vi "Singing Helmet.vi"(8 "error in (no error)":errorcluster) -> (0 "error out":errorcluster)   [LabVIEW 2020, in "MainVIs.lvlib"]
doc: "This template is for the Queued Message Handler design pattern.\n\nThe Event Handling Loop generates messages based on user interface actions.\n\nThe Message Handling Loop processes messages generated by the Event Handling Loop, or by other messages. The messages are string values, so new messages can be added easily to the Message Cases case structure in the Message Handling Loop. Each message cluster can also provide an optional value for Message Data, which is a variant that can be converted to whatever message-specific data is required."
uses:
  MainVIs.lvlib
  Collection Support/Controls/UI Data SH.ctl
  Collection Support/Controls/CollectStates.ctl
  Collection Support/Controls/FirstCall.ctl
  Collection Support/Message Queue/Enqueue Message (Single).vi
  Collection Support/Message Queue/Enqueue Message (Array).vi
  <vilib>/Utility/error.llb/Error Cluster From Error Code.vi
  <vilib>/ErrorRing/Error Ring.xnode
  Collection Support/Message Queue/Message Queue.lvlib
  Collection Support/User Event - Stop/User Event - Stop.lvlib
  CollectionSupport.lvlib
panel:
  out "Flow":dbl
  out "Pressure":dbl
  in  "Blank Button":bool
  in  "Calibrate":bool
  out "Message":string
  in  "Settings":bool
  in  "Collect":bool
  in  "Exit":bool
  out "Pressure":dynamicdata(graph)
  out "Audio Chart":dynamicdata(graph)
  out "Flow":dynamicdata(graph)
  out "All Data Collected":dynamicdata(graph)
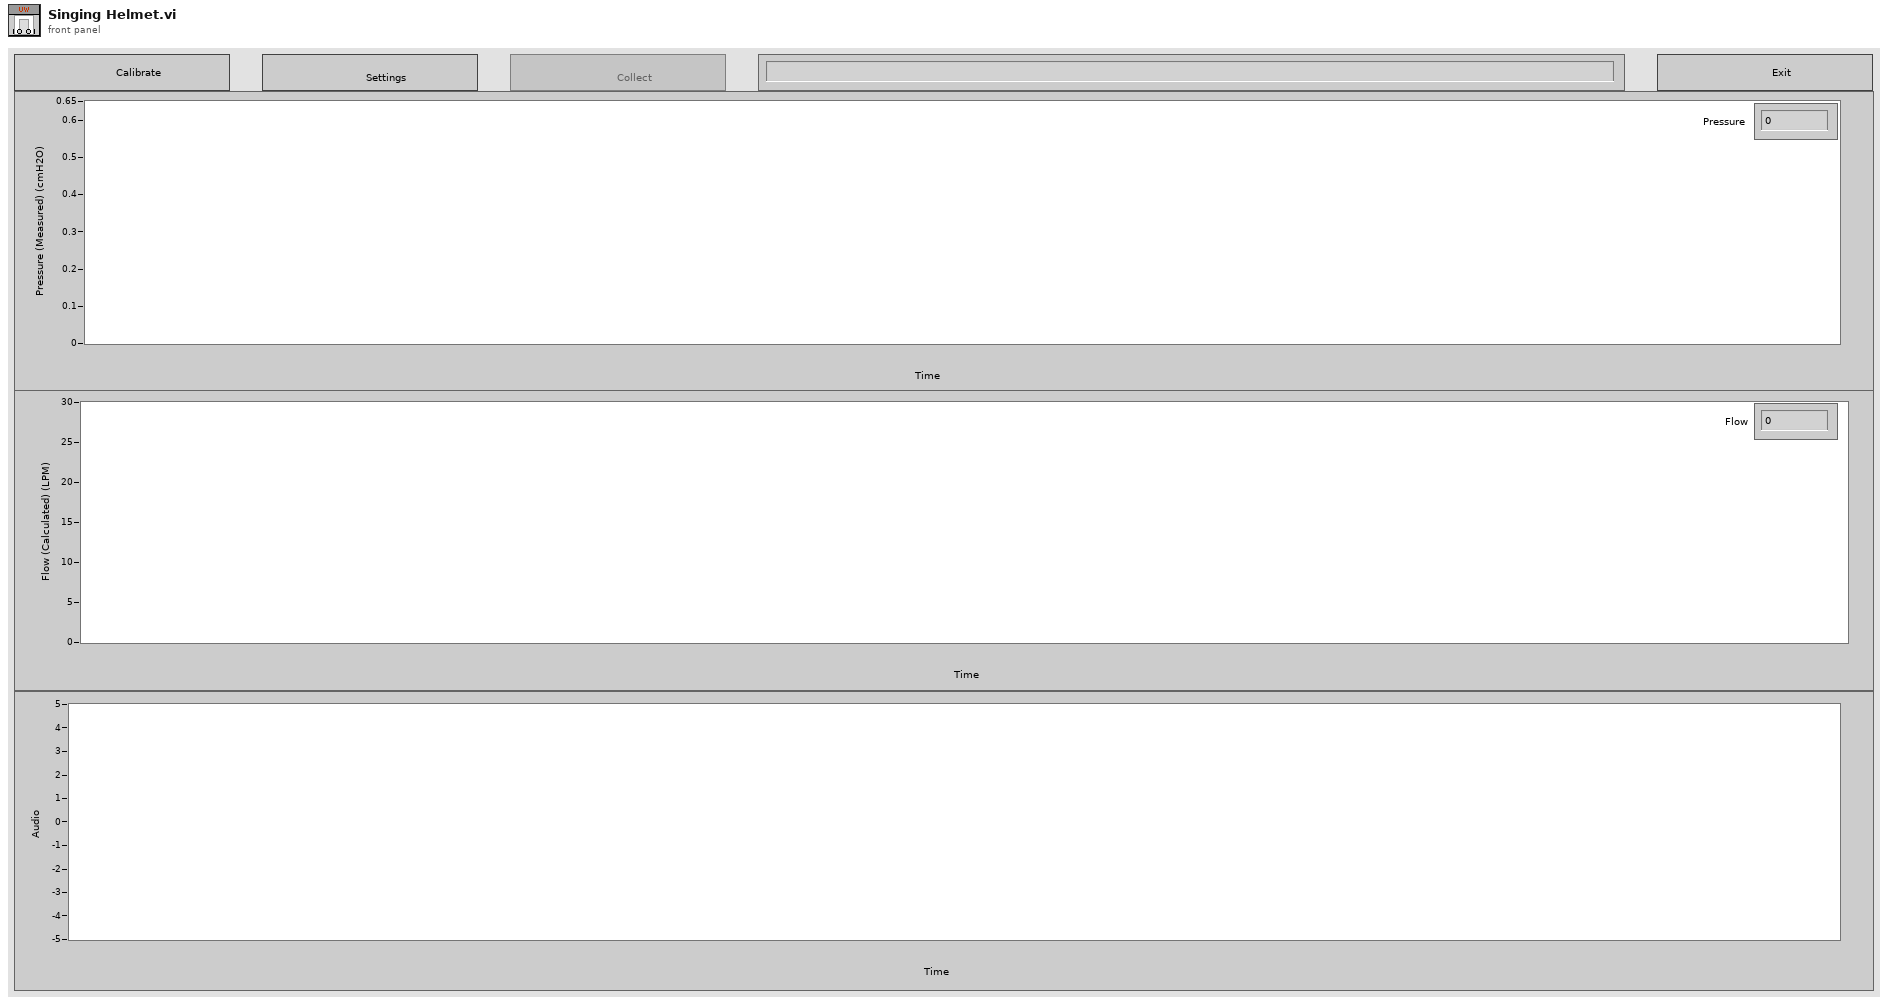
[diagram p1: front panel]
types:
  T1 = typedef "CollectionSupport.lvlib/UI Data SH.ctl" = cluster{"Message":string, "Trial":i32, "Calibrate Ref":refnum<vi>, "Collect Ref":refnum<vi>, "Exit Button Ref":refnum<vi>, "Settings Ref":refnum<vi>, "Data Display Ref":refnum<vi>, "Time":dbl, "Slope":dbl, "Intercept":dbl, "Gain":dbl, "Offset":dbl, "Task":string, "Subject":string, "Pressure":dynamicdata, "Flow":dynamicdata, "Audio Chart":dynamicdata, "Pressure/Flow":dynamicdata, "Audio Collected":dynamicdata}
  T2 = typedef "CollectionSupport.lvlib/Message Queue.lvlib/All Message Queues.ctl" = cluster{"UI":refnum<queue>}
  T3 = typedef "CollectionSupport.lvlib/CollectStates.ctl" = enum16{"Start", "Run", "Save", "Check", "Exit"}
  T4 = typedef "CollectionSupport.lvlib/FirstCall.ctl" = enum16{"First", "After"}
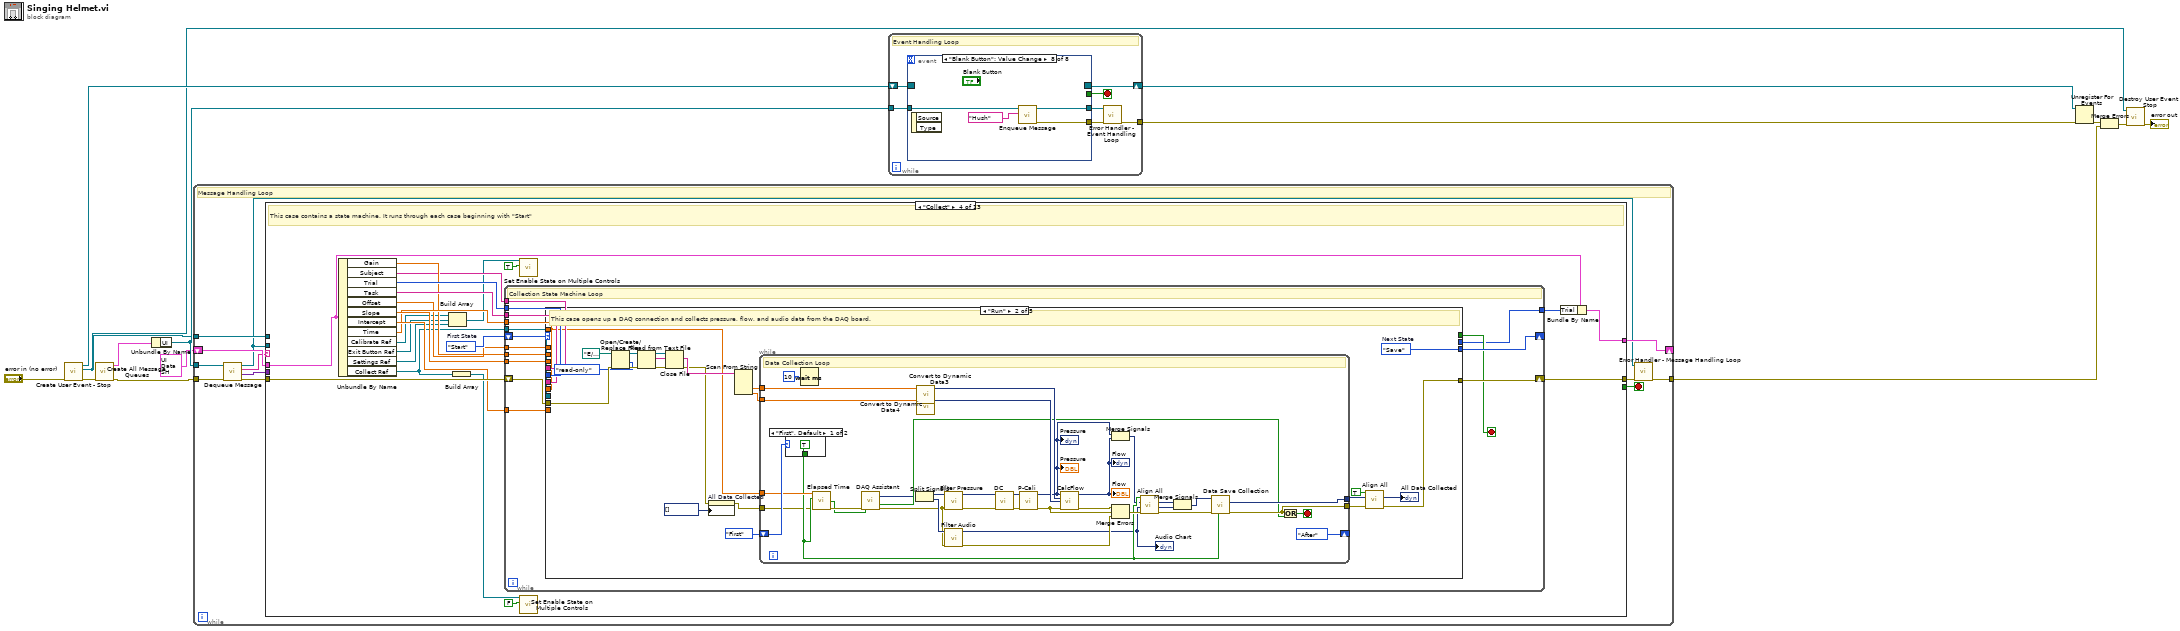
[diagram p0: block diagram]
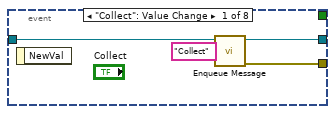
[diagram p2: hidden frame]
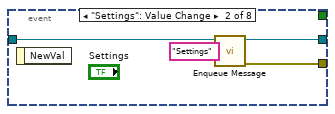
[diagram p3: hidden frame]
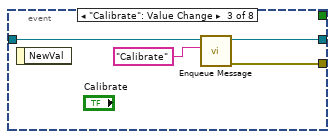
[diagram p4: hidden frame]
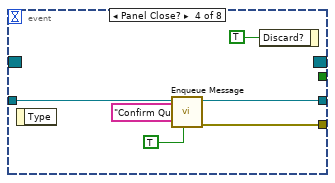
[diagram p5: hidden frame]
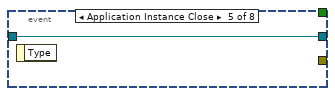
[diagram p6: hidden frame]
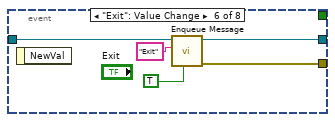
[diagram p7: hidden frame]
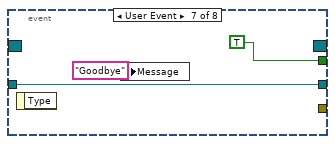
[diagram p8: hidden frame]
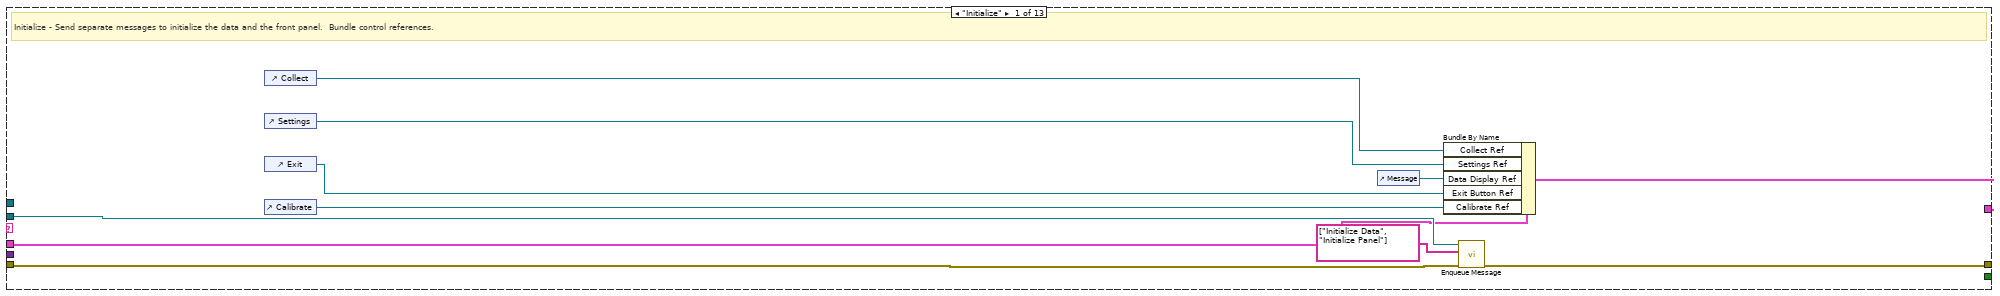
[diagram p9: hidden frame]
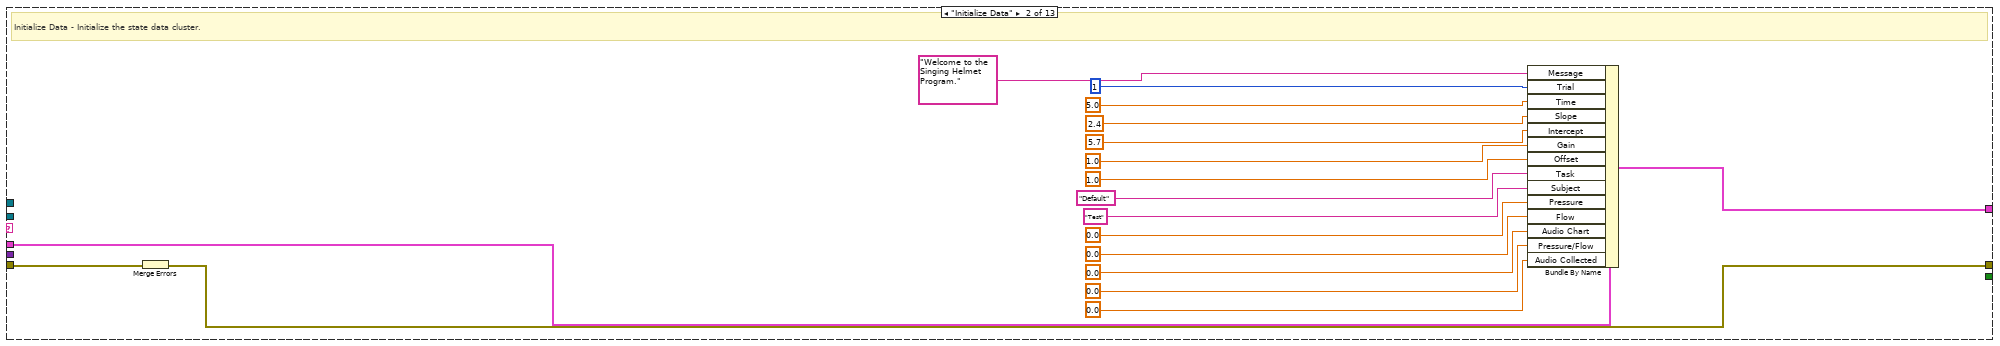
[diagram p10: hidden frame]
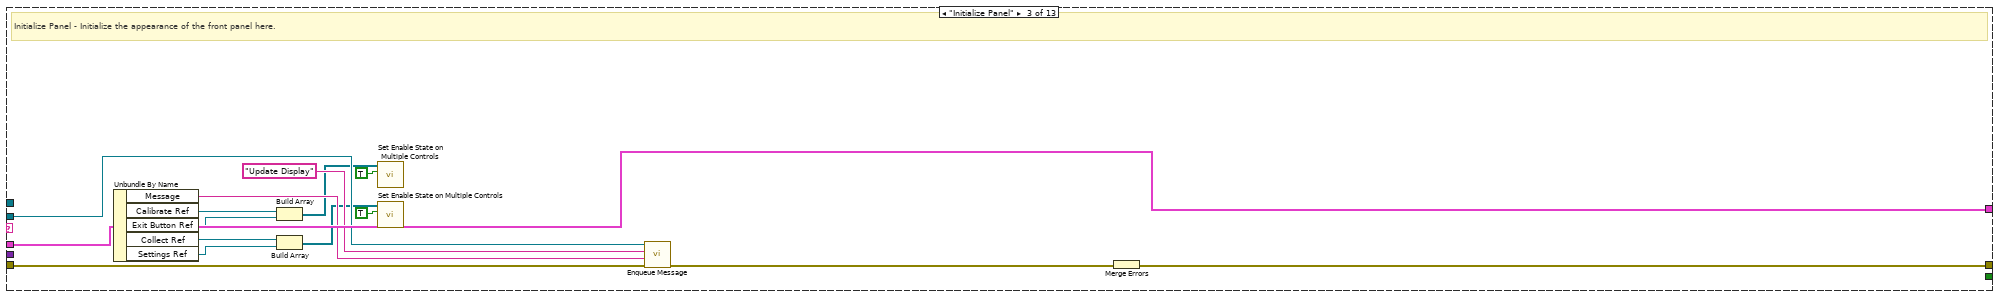
[diagram p11: hidden frame]
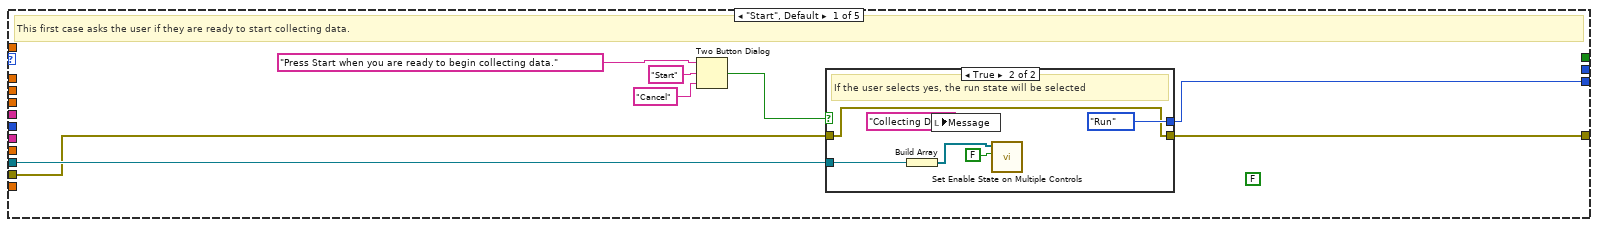
[diagram p12: hidden frame]
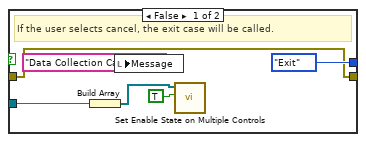
[diagram p13: hidden frame]
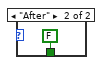
[diagram p14: hidden frame]
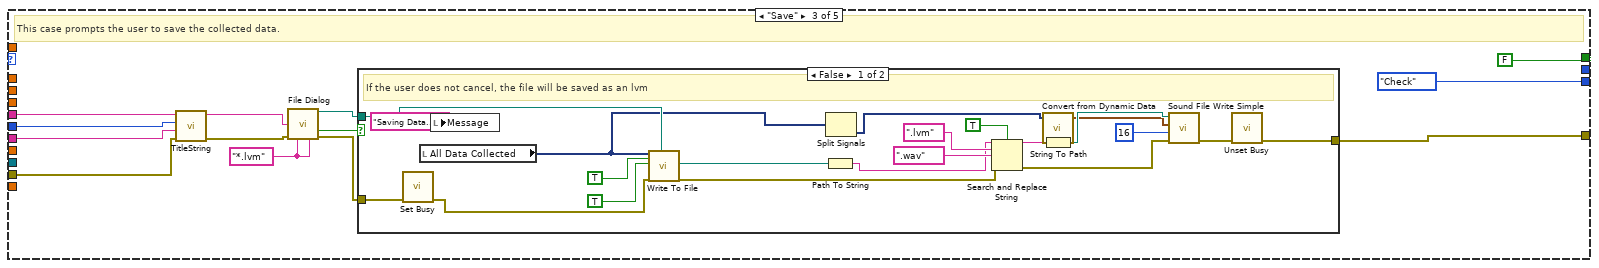
[diagram p15: hidden frame]
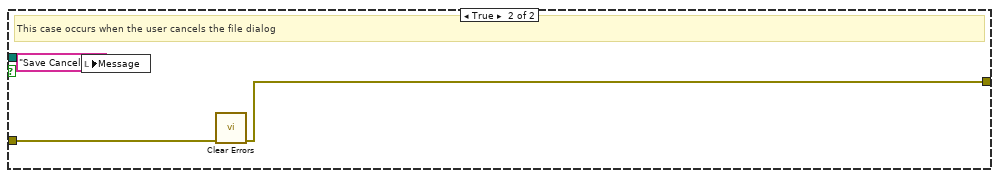
[diagram p16: hidden frame]
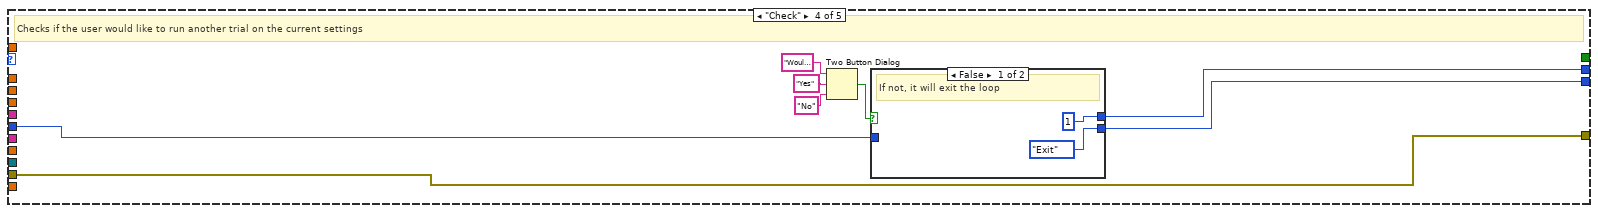
[diagram p17: hidden frame]
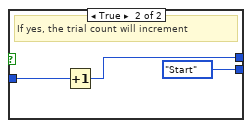
[diagram p18: hidden frame]
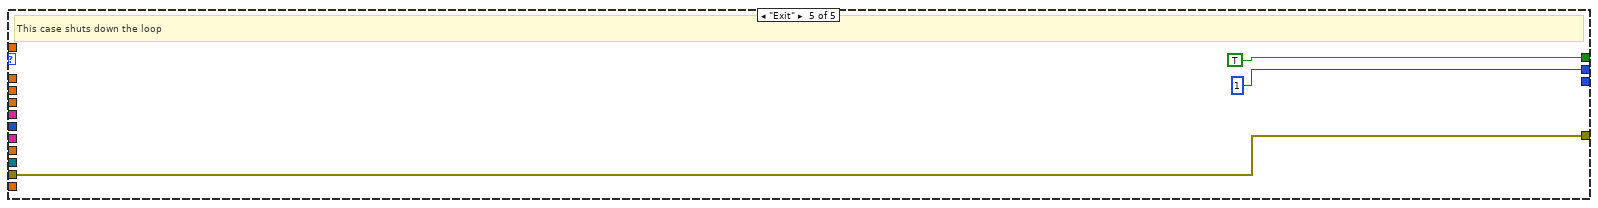
[diagram p19: hidden frame]
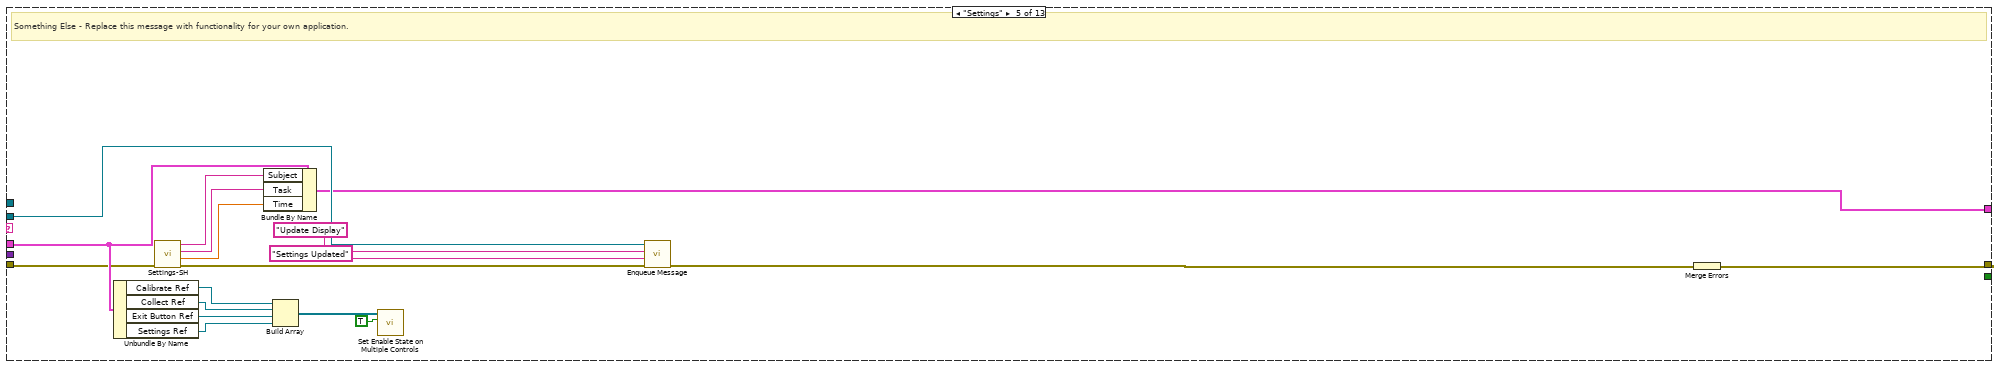
[diagram p20: hidden frame]
diagram:
  n1 = call "Create User Event - Stop.vi"("error in (no error)"="error in (no error)") -> ("error out"=w9:errorcluster, "User Event - Stop"=w7:refnum<user-event>, "Stop Event Registration Refnum"=w10:refnum<event-registration>)  [unwired: 8 in]
  n2 = call "Create All Message Queues.vi"("error in (no error)"=w9) -> ("error out"=w14:errorcluster, "Message Queues out"=w13:T2)  [unwired: 9 in]
  n3 = Unbundle By Name(w13) -> ("UI"=w11:refnum<queue>)
  n4 = while {
    tunnel: w11 -> [w18]
    shift-right: [w25] -> _
    shift-left: T1 {"Message"="", "Trial"=0, "Calibrate Ref"=refnum, "Collect Ref"=refnum, "Exit Button Ref"=refnum, "Settings Ref"=refnum, "Data Display Ref"=refnum, "Time"=0.0, "Slope"=0.0, "Intercept"=0.0, "Gain"=0.0, "Offset"=0.0, "Task"="", "Subject"="", "Pressure"=[], "Flow"=[], "Audio Chart"=[], "Pressure/Flow"=[], "Audio Collected"=[]} ("UI Data") -> [w26]
    tunnel: w7 -> [w23]
    tunnel: w14 -> [w22]
    tunnel: [w16] -> w12
    stop <- w24 stop-if-true
    # "Message Handling Loop"
    n5 = call "Dequeue Message.vi"("error in (no error)"=w22, "Message Queue"=w18) -> ("error out"=w21:errorcluster, "Message Data"=w19:variant, "Message"=w20:string, "dup Message Queue"=w17:refnum<queue>)  [unwired: 6 in]
    n6 = case "Message Cases" shown="\"Collect\"" w20 {
      selector: w20 -> [_ _ _ _ _ _ _ _ _ _ _ _ w314]
      tunnel: w17 -> [w35 _ w67 _ w255 w272 _ _ w287 w298 _ w313 _]
      tunnel: w21 -> [w36 w55 w68 w91 w244 w273 w276 w282 w295 w302 w305 w308 _]
      tunnel: [w37 w51 w69 w82 w257 w263 w276 w283 w288 w300 w303 w309 w315] -> w15
      tunnel: w26 -> [w34 w54 w70 w81 w251 w260 w277 w284 w294 w301 w304 w312 w316]
      tunnel: [w33 w53 w70 w80 w252 w259 w277 w284 w294 w301 w304 w312 w316] -> w25
      tunnel: [_ _ _ _ _ _ _ _ _ _ _ TRUE _] -> w24
      tunnel: w19 -> [_ _ _ _ _ _ _ w281 w293 _ _ _ _]
      tunnel: w23 -> [_ _ _ _ _ _ _ _ _ _ _ w307 _]
      frame "Initialize" {
        # "Initialize - Send separate messages to initialize the data and the front panel.  Bundle control references."
        n7 = control-ref of="Collect"() -> (w32:refnum<vi>)
        n8 = control-ref of="Settings"() -> (w31:refnum<vi>)
        n9 = control-ref of="Exit"() -> (w29:refnum<vi>)
        n10 = control-ref of="Calibrate"() -> (w27:refnum<vi>)
        n11 = control-ref of="Message"() -> (w30:refnum<vi>)
        n12 = Bundle By Name(cluster=w34, "Collect Ref"=w32, "Settings Ref"=w31, "Data Display Ref"=w30, "Exit Button Ref"=w29, "Calibrate Ref"=w27) -> (w33:T1)
        n13 = call-poly "Enqueue Message.vi"("error in (no error)"=w36, "Message Array"=string[] ["Initialize Data", "Initialize Panel"], "Message Queue"=w35) -> ("error out"=w37:errorcluster)  [unwired: 7 in, 1 out]
      }
      frame "Initialize Data" {
        # "Initialize Data - Initialize the state data cluster."
        n14 = Merge Errors(w55) -> (w51:errorcluster)
        n15 = Bundle By Name(cluster=w54, "Message"="Welcome to the Singing Helmet Program." ("Initial Message"), "Trial"=1, "Time"=5.0, "Slope"=2.4, "Intercept"=5.7, "Gain"=1.0, "Offset"=1.0, "Task"="Default", "Subject"="Test", "Pressure"=0.0, "Flow"=0.0, "Audio Chart"=0.0, "Pressure/Flow"=0.0, "Audio Collected"=0.0) -> (w53:T1)
      }
      frame "Initialize Panel" {
        # "Initialize Panel - Initialize the appearance of the front panel here."
        n16 = Unbundle By Name(w70) -> ("Message"=w64:string, "Calibrate Ref"=w61:refnum<vi>, "Exit Button Ref"=w58:refnum<vi>, "Collect Ref"=w57:refnum<vi>, "Settings Ref"=w56:refnum<vi>)
        n17 = Build Array(w61, w58) -> (w62:refnum<vi>[])
        n18 = Build Array(w57, w56) -> (w59:refnum<vi>[])
        n19 = call "Set Enable State on Multiple Controls.vi"("Enable?"=TRUE, "Controls"=w62) -> ()  [unwired: 10 in]
        n20 = call "Set Enable State on Multiple Controls.vi"("Enable?"=TRUE, "Controls"=w59) -> ()  [unwired: 10 in]
        n21 = call-poly "Enqueue Message.vi"("error in (no error)"=w68, "Message Data"=w64, "Message"="Update Display", "Message Queue"=w67) -> ("error out"=w66:errorcluster)  [unwired: 6 in, 1 out]
        n22 = Merge Errors(w66) -> (w69:errorcluster)
      }
      frame "Collect" {
        w92 = CollectStates."Start"  # First State
        # "This case contains a state machine. It runs through each case beginning with \"Start\""
        n23 = Unbundle By Name(w81) -> ("Gain"=w84:dbl, "Subject"=w83:string, "Trial"=w85:i32, "Task"=w86:string, "Offset"=w87:dbl, "Slope"=w90:dbl, "Intercept"=w89:dbl, "Time"=w88:dbl, "Calibrate Ref"=w76:refnum<vi>, "Exit Button Ref"=w75:refnum<vi>, "Settings Ref"=w74:refnum<vi>, "Collect Ref"=w71:refnum<vi>)
        n24 = Build Array(w76, w75, w74) -> (w72:refnum<vi>[])
        n25 = Build Array(w71) -> (w73:refnum<vi>[])
        n26 = while {
          tunnel: w88 -> [w93]
          shift-right: [w102] -> w82
          shift-left: w91 -> [w107]
          tunnel: w89 -> [w106]
          tunnel: w90 -> [w105]
          tunnel: w84 -> [w104]
          tunnel: w87 -> [w103]
          shift-right: [w100] -> _
          shift-left: w92 -> [w101]
          tunnel: w85 -> [w98]
          tunnel: w83 -> [w97]
          tunnel: w86 -> [w96]
          tunnel: [w95] -> w79
          tunnel: w71 -> [w94]
          stop <- w99 stop-if-true
          # "Collection State Machine Loop"
          n27 = case shown="\"Run\"" w101 {
            tunnel: w107 -> [w109 w147 w189 w228 w239]
            tunnel: w93 -> [_ _ _ _ _]
            tunnel: w106 -> [_ _ _ _ _]
            tunnel: w105 -> [_ _ _ _ _]
            tunnel: w104 -> [_ _ _ _ _]
            tunnel: w103 -> [_ _ _ _ _]
            tunnel: [w108 w132 w196 w228 w239] -> w102
            tunnel: [w111 w148 CollectStates."Check" w226 _] -> w100
            tunnel: [_ _ FALSE _ TRUE] -> w99
            tunnel: w98 -> [_ _ w193 w225 _]
            tunnel: w97 -> [_ _ w192 _ _]
            tunnel: w96 -> [_ _ w191 _ _]
            tunnel: [_ _ _ w224 1] -> w95
            tunnel: w94 -> [w110 _ _ _ _]
            tunnel: w93 -> [_ w136 _ _ _]
            frame "Start", Default {
              (unwired) FALSE ("Value (Signaling)")
              # "This first case asks the user if they are ready to start collecting data."
              n28 = Two Button Dialog(message="Press Start when you are ready to begin collecting data.", 1:"Cancel" ("F button name (\"Cancel\")"), 2:"Start" ("T button name (\"OK\")")) -> (T button?=w112:bool)
              n29 = case shown="True" w112 {
                tunnel: [CollectStates."Exit" CollectStates."Run"] -> w111
                tunnel: w110 -> [w118 w123]
                tunnel: w109 -> [w116 w122]
                tunnel: [w116 w122] -> w108
                frame False {
                  # "If the user selects cancel, the exit case will be called."
                  n30 = Build Array(w118) -> (w119:refnum<vi>[])
                  n31 = local write "Message"("Data Collection Cancelled" ("Message")) -> ()
                  n32 = call "Set Enable State on Multiple Controls.vi"("Enable?"=TRUE, "Controls"=w119) -> ()  [unwired: 10 in]
                }
                frame True {
                  # "If the user selects yes, the run state will be selected"
                  n33 = Build Array(w123) -> (w126:refnum<vi>[])
                  n34 = local write "Message"("Collecting Data" ("Message")) -> ()
                  n35 = call "Set Enable State on Multiple Controls.vi"("Enable?"=FALSE, "Controls"=w126) -> ()  [unwired: 10 in]
                }
              }
            }
            frame "Run" {
              w148 = CollectStates."Save"  # Next State
              # "This case opens up a DAQ connection and collects pressure, flow, and audio data from the DAQ board."
              n36 = Open/Create/Replace File(file path (use dialog)=path "E:/Program Files/Master Aero Program/Calibration .txt files/SH Cali.txt", error in=w147, access (0:read/write)=enum16{"read/write", "read-only", "write-only"}."read-only") -> (refnum out=w141:refnum<file>, error out=w143:errorcluster)  [unwired: 3 in, 1 out]
              n37 = Read from Text File(file (use dialog)=w141, error in=w143) -> (refnum out=w140:refnum<file>, text=w142:string, error out=w144:errorcluster)  [unwired: 2 in, 1 out]
              n38 = Close File(refnum=w140, error in=w144) -> (error out=w128:errorcluster)  [unwired: 1 out]
              n39 = property on="All Data Collected" class="WFChart (strict)"(error in=w128, "History Data"=dynamicdata[] []) -> (error out=w129:errorcluster)  [unwired: 1 in, 1 out]
              n40 = Scan From String(input string=w142) -> (output 1=w146:dbl, output 2=w145:dbl)  [unwired: 5 in, 3 out]
              n41 = while {
                tunnel: w146 -> [w183]
                tunnel: w145 -> [w184]
                tunnel: [w167] -> w135
                tunnel: [w166] -> w134
                shift-right: [FirstCall."After"] -> _
                shift-left: FirstCall."First" -> [w163]
                tunnel: w136 -> [w160]
                tunnel: w129 -> [w149]
                stop <- w179 stop-if-true
                # "Data Collection Loop"
                n42 = case shown="\"First\", Default" w163 {
                  tunnel: [TRUE FALSE] -> w153
                  frame "First", Default {
                  }
                  frame "After" {
                  }
                }
                n43 = Wait (ms)(milliseconds to wait=u32 10) -> ()  [unwired: 1 out]
                n44 = call "Elapsed Time"("Time Target (s)"=w160, "Reset"=w153, "error in (no error)"=w149) -> ("Time has Elapsed"=w161:bool, "error out"=w162:errorcluster)  [unwired: 9 in, 6 out]
                n45 = call "DAQ Assistant"("error in"=w162, "stop (F)"=w161) -> ("data"=w157:dynamicdata, "stopped"=w159:bool, "error out"=w158:errorcluster)  [unwired: 14 in, 1 out]
                n46 = Split Signals(w157) -> (w182:dynamicdata, w181:dynamicdata)  [unwired: 2 in]
                n47 = call "Convert to Dynamic Data3"("Double"=w183) -> ("Dynamic Data Type"=w173:dynamicdata)  [unwired: 3 in]
                n48 = call "Convert to Dynamic Data4"("Double"=w184) -> ("Dynamic Data Type"=w174:dynamicdata)  [unwired: 3 in]
                n49 = call "Filter Pressure"("error in (no error)"=w158, "Signal"=w182) -> ("error out"=w178:errorcluster, "Filtered Signal"=w177:dynamicdata)  [unwired: 8 in]
                n50 = call "Filter Audio"("error in (no error)"=w158, "Signal"=w181) -> ("error out"=w171:errorcluster, "Filtered Signal"=w151:dynamicdata)  [unwired: 8 in]
                "Audio Chart" <- w151
                n51 = call "DC"("Signals"=w177, "error in (no error)"=w178) -> ("Mean (DC)"=w176:dynamicdata, "error out"=w175:errorcluster)  [unwired: 12 in]
                n52 = call "P-Cali.vi"("V"=w176, "error in (no error)"=w175) -> ("Result"=w155:dynamicdata, "error out"=w169:errorcluster)  [unwired: 12 in]
                "Pressure" <- w155
                "Pressure" <- w155
                n53 = call "CalcFlow.vi"("Pressure"=w155, "Slope"=w173, "Intercept"=w174, "error in (no error)"=w169) -> ("Result"=w154:dynamicdata, "error out"=w170:errorcluster)  [unwired: 10 in]
                "Flow" <- w154
                "Flow" <- w154
                n54 = Merge Signals(w155, w154) -> (w152:dynamicdata)
                n55 = Merge Errors(w170, w169, w171) -> (w172:errorcluster)
                n56 = call "Align All"("error in (no error)"=w172, "Signals 2"=w151, "Signals"=w152, "Reset"=w153) -> ("error out"=w168:errorcluster, "Resampled Signals 2"=w150:dynamicdata, "Resampled Signals"=w156:dynamicdata)  [unwired: 5 in]
                n57 = Merge Signals(w156, w150) -> (w165:dynamicdata)
                n58 = call "Data Save Collection"("Reset"=w153, "error in (no error)"=w168, "Signals"=w165) -> ("error out"=w167:errorcluster, "Collected Signals"=w166:dynamicdata)  [unwired: 7 in]
                n59 = Or(x=w167, y=w159) -> (x .or. y?=w179:bool)
              }
              n60 = call "Align All"("error in (no error)"=w135, "Signals"=w134, "Reset"=TRUE) -> ("error out"=w132:errorcluster, "Resampled Signals"=→"All Data Collected":dynamicdata)  [unwired: 6 in, 1 out]
            }
            frame "Save" {
              w187 = "*.lvm" ("pattern label")
              # "This case prompts the user to save the collected data."
              n61 = call "TitleString.vi"("error in"=w189, "Task"=w191, "Trial"=w193, "Subject"=w192) -> ("error out"=w188:errorcluster, "String"=w190:string)  [unwired: 6 in]
              n62 = call "File Dialog"("default name"=w190, "error in"=w188, "pattern (all files)"=w187, "pattern label"=w187) -> ("selected path"=w195:path, "cancelled"=w194:bool, "error out"=w197:errorcluster)  [unwired: 8 in, 1 out]
              n63 = case shown="False" w194 {
                tunnel: w197 -> [w209 w222]
                tunnel: [w206 w221] -> w196
                tunnel: w195 -> [w220 _]
                frame False {
                  # "If the user does not cancel, the file will be saved as an lvm"
                  n64 = call <vilib>:"Set Busy.vi"("error in (no error)"=w209) -> ("error out"=w208:errorcluster)  [unwired: 9 in, 1 out]
                  n65 = local read "All Data Collected"() -> (w204:dynamicdata)
                  n66 = local write "Message"("Saving Data..." ("Message")) -> ()
                  n67 = call "Write To File"("Signals"=w204, "Reset"=TRUE, "Enable"=TRUE, "error in (no error)"=w208, "Filename"=w220) -> ("Filename Out"=w212:path, "error out"=w215:errorcluster)  [unwired: 12 in, 1 out]
                  n68 = Path To String(path=w212) -> (string=w213:string)
                  n69 = Split Signals(w204) -> (w203:dynamicdata)  [unwired: 3 in, 2 out]
                  n70 = Search and Replace String(case sensitive?=TRUE ("ignore case? (F)"), input string=w213, search string=".lvm", replace string=".wav" ("replace string (\"\")"), error in=w215) -> (result string=w211:string, error out=w216:errorcluster)  [unwired: 3 in, 2 out]
                  n71 = call "Convert from Dynamic Data"("Dynamic Data Type"=w203) -> ("Array of Waveform"=w210:waveform(dbl)[])  [unwired: 3 in]
                  n72 = String To Path(string=w211) -> (path=w217:path)
                  n73 = call <vilib>:"Sound File Write Simple.vi"("error in (no error)"=w216, "bits per sample"=16, "data"=w210, "path"=w217) -> ("error out"=w207:errorcluster)  [unwired: 6 in, 1 out]
                  n74 = call <vilib>:"Unset Busy.vi"("error in (no error)"=w207) -> ("error out"=w206:errorcluster)  [unwired: 10 in]
                }
                frame True {
                  # "This case occurs when the user cancels the file dialog"
                  n75 = local write "Message"("Save Cancelled." ("Message 2")) -> ()
                  n76 = call <vilib>:"Clear Errors.vi"("error in (no error)"=w222) -> ("error out"=w221:errorcluster)  [unwired: 5 in, 1 out]
                }
              }
            }
            frame "Check" {
              # "Checks if the user would like to run another trial on the current settings"
              n77 = Two Button Dialog(message="Would you like to run another trial?", 1:"No" ("F button name (\"Cancel\")"), 2:"Yes" ("T button name (\"OK\")")) -> (T button?=w227:bool)
              n78 = case shown="False" w227 {
                tunnel: [CollectStates."Exit" CollectStates."Start"] -> w226
                tunnel: w225 -> [_ w235]
                tunnel: [1 w234] -> w224
                frame False {
                  # "If not, it will exit the loop"
                }
                frame True {
                  # "If yes, the trial count will increment"
                  n79 = Increment(x=w235) -> (x+1=w234:i32)
                }
              }
            }
            frame "Exit" {
              # "This case shuts down the loop"
            }
          }
        }
        n80 = call "Set Enable State on Multiple Controls.vi"("Enable?"=TRUE, "Controls"=w72) -> ()  [unwired: 10 in]
        n81 = call "Set Enable State on Multiple Controls.vi"("Enable?"=FALSE, "Controls"=w73) -> ()  [unwired: 10 in]
        n82 = Bundle By Name(cluster=w81, "Trial"=w79) -> (w80:T1)
      }
      frame "Settings" {
        # "Something Else - Replace this message with functionality for your own application."
        n83 = Unbundle By Name(w251) -> ("Calibrate Ref"=w248:refnum<vi>, "Collect Ref"=w246:refnum<vi>, "Exit Button Ref"=w247:refnum<vi>, "Settings Ref"=w245:refnum<vi>)
        n84 = call "Settings-SH.vi"("Error In"=w244) -> ("error out"=w243:errorcluster, "Time Target (sec)"=w240:dbl, "Task"=w241:string, "Subject"=w242:string)  [unwired: 7 in]
        n85 = Bundle By Name(cluster=w251, "Subject"=w242, "Task"=w241, "Time"=w240) -> (w252:T1)
        n86 = Build Array(w248, w246, w247, w245) -> (w249:refnum<vi>[])
        n87 = call "Set Enable State on Multiple Controls.vi"("Enable?"=TRUE, "Controls"=w249) -> ()  [unwired: 10 in]
        n88 = call-poly "Enqueue Message.vi"("error in (no error)"=w243, "Message Data"="Settings Updated" ("\"Do Something Else\" button pressed"), "Message"="Update Display", "Message Queue"=w255) -> ("error out"=w256:errorcluster)  [unwired: 6 in, 1 out]
        n89 = Merge Errors(w256) -> (w257:errorcluster)
      }
      frame "Calibrate" {
        # "This case opens the calibration SubVI"
        n90 = Unbundle By Name(w260) -> ("Collect Ref"=w267:refnum<vi>, "Calibrate Ref"=w266:refnum<vi>, "Exit Button Ref"=w265:refnum<vi>, "Settings Ref"=w264:refnum<vi>)
        n91 = Build Array(w266, w265, w264) -> (w269:refnum<vi>[])
        n92 = Build Array(w267) -> (w268:refnum<vi>[])
        n93 = call "Set Enable State on Multiple Controls.vi"("Enable?"=TRUE, "Controls"=w268) -> ()  [unwired: 10 in]
        n94 = call "Set Enable State on Multiple Controls.vi"("Enable?"=TRUE, "Controls"=w269) -> ()  [unwired: 10 in]
        n95 = call-poly "Enqueue Message.vi"("error in (no error)"=w273, "Message Data"="Opening Calibration" ("\"Do Something Else\" button pressed"), "Message"="Update Display", "Message Queue"=w272) -> ("error out"=w258:errorcluster)  [unwired: 6 in, 1 out]
        n96 = call "Calibration-SH.vi"("Error In"=w258) -> ("Error Out"=w263:errorcluster, "Offset"=w261:dbl, "Gain"=w262:dbl)  [unwired: 8 in]
        n97 = Bundle By Name(cluster=w260, "Gain"=w262, "Offset"=w261) -> (w259:T1)
      }
      frame "Hush" {
        # "!"
      }
      frame "Update Display" {
        # "Update Display - Convert the message data to a string to display in the Data Display indicator."
        n98 = Variant To Data(error in=w282, type="", Variant=w281) -> (data=→"Message":string, error out=w279:errorcluster)
        n99 = Merge Errors(w279) -> (w283:errorcluster)
      }
      frame "Error" {
        # "Error - Check the error message data and respond accordingly. This message is sent by the \"Error Handler\" VIs at the end of each loop in this application."
        n100 = Variant To Data(error in=w295, type=errorcluster {"status"=FALSE, "code"=0, "source"=""} ("error constant"), Variant=w293) -> (data=w291:errorcluster, error out=w290:errorcluster)
        n101 = call-poly "Enqueue Message.vi"("Priority Message? (F)"=TRUE, "Message"="Exit", "Message Queue"=w287) -> ("error out"=w289:errorcluster)  [unwired: 7 in, 1 out]
        n102 = call <vilib>:"Simple Error Handler.vi"("error in (no error)"=w291) -> ()  [unwired: 4 in, 5 out]
        n103 = Merge Errors(w289, w290) -> (w288:errorcluster)
      }
      frame "Confirm Quit" {
        # "Confirm Quit - Message that can confirm whether or not the user wants to exit the application."
        n104 = call-poly "Enqueue Message.vi"("Priority Message? (F)"=TRUE, "error in (no error)"=w302, "Message"="Exit", "Message Queue"=w298) -> ("error out"=w299:errorcluster)  [unwired: 6 in, 1 out]
        n105 = Merge Errors(w299) -> (w300:errorcluster)
      }
      frame "---Copy This Frame---" {
        # "Duplicate this frame when creating new messages.  Change this comment in the duplicated frame to describe this message."
        n106 = Merge Errors(w305) -> (w303:errorcluster)
      }
      frame "Exit" {
        # "Exit - Exit the application."
        n107 = Release Queue(queue=w313, error in (no error)=w308) -> (error out=w310:errorcluster)  [unwired: 1 in, 2 out]
        n108 = call "Fire User Event - Stop.vi"("User Event - Stop"=w307) -> ("error out"=w306:errorcluster)  [unwired: 10 in]
        n109 = Merge Errors(w306, w310) -> (w309:errorcluster)
      }
      frame Default {
        # "'Default' case only runs if there is a message that isn't defined in any of the other cases.  Output a programming error."
        n110 = xnode "Error Ring"("parameter 0"=w314) -> ("error out"=w315:errorcluster)
      }
    }
    n111 = call "Error Handler - Message Handling Loop.vi"("error in (no error)"=w15, "Message Queue"=w17) -> ("dup error in"=w16:errorcluster)  [unwired: 8 in, 1 out]
  }
  n112 = while {
    tunnel: w11 -> [w330]
    shift-right: [w328] -> w5
    shift-left: w10 -> [w329]
    tunnel: [w324] -> w4
    stop <- w326 stop-if-true
    # "Event Handling Loop"
    n113 = event shown="[7] \"Blank Button\": Value Change" {
      selector: w329 -> [_ _ _ _ _ _ _ _]
      dyn-events: [_ _ _ _ _ _ _ _] -> w328
      timeout: _ -> [_ _ _ _ _ _ _ _]
      tunnel: [_ _ _ _ _ _ TRUE ("Discard?") _] -> w326
      tunnel: w330 -> [w334 w338 w341 w347 w349 w354 w357 w360]
      tunnel: [w331 w335 w339 w346 _ w353 _ w358] -> w327
      tunnel: [w333 w337 w340 w345 w349 w352 w357 w359] -> w325
      event "Collect": Value Change {
        n114 = event-data() -> ()  [unwired: 1 in, 1 out]
        n115 = call-poly "Enqueue Message.vi"("Message"="Collect", "Message Queue"=w334) -> ("error out"=w331:errorcluster, "dup Message Queue"=w333:refnum<queue>)  [unwired: 8 in]
      }
      event "Settings": Value Change {
        n116 = event-data() -> ()  [unwired: 1 in, 1 out]
        n117 = call-poly "Enqueue Message.vi"("Message"="Settings", "Message Queue"=w338) -> ("error out"=w335:errorcluster, "dup Message Queue"=w337:refnum<queue>)  [unwired: 8 in]
      }
      event "Calibrate": Value Change {
        n118 = event-data() -> ()  [unwired: 1 in, 1 out]
        n119 = call-poly "Enqueue Message.vi"("Message"="Calibrate", "Message Queue"=w341) -> ("error out"=w339:errorcluster, "dup Message Queue"=w340:refnum<queue>)  [unwired: 8 in]
      }
      event Panel Close? {
        n120 = event-data() -> ()  [unwired: 1 in, 1 out]
        n121 = call-poly "Enqueue Message.vi"("Priority Message? (F)"=TRUE, "Message"="Confirm Quit", "Message Queue"=w347) -> ("error out"=w346:errorcluster, "dup Message Queue"=w345:refnum<queue>)  [unwired: 7 in]
        n122 = event-data("Discard?"=TRUE) -> ()  [unwired: 1 in, 1 out]
      }
      event Application Instance Close {
        n123 = event-data() -> ()  [unwired: 1 in, 1 out]
      }
      event "Exit": Value Change {
        n124 = event-data() -> ()  [unwired: 1 in, 1 out]
        n125 = call-poly "Enqueue Message.vi"("Priority Message? (F)"=TRUE, "Message"="Exit", "Message Queue"=w354) -> ("error out"=w353:errorcluster, "dup Message Queue"=w352:refnum<queue>)  [unwired: 7 in]
      }
      event User Event {
        n126 = event-data() -> ()  [unwired: 1 in, 1 out]
        n127 = local write "Message"("Goodbye" ("VI Stopped")) -> ()
      }
      event "Blank Button": Value Change {
        n128 = event-data() -> ()  [unwired: 1 in, 2 out]
        n129 = call-poly "Enqueue Message.vi"("Message"="Hush", "Message Queue"=w360) -> ("error out"=w358:errorcluster, "dup Message Queue"=w359:refnum<queue>)  [unwired: 8 in]
      }
    }
    n130 = call "Error Handler - Event Handling Loop.vi"("error in (no error)"=w327, "Message Queue"=w325) -> ("dup error in"=w324:errorcluster)  [unwired: 8 in, 1 out]
  }
  n131 = Unregister For Events(event registration refnum=w5, error in=w4) -> (error out=w6:errorcluster)
  n132 = Merge Errors(w6, w12) -> (w8:errorcluster)
  n133 = call "Destroy User Event - Stop.vi"("error in (no error)"=w8, "User Event - Stop"=w7) -> ("error out"=→"error out":errorcluster)  [unwired: 9 in]
